vi "CompressAndUpdate(NumericArray).vi"(7 "force CVT update (false)":bool, 8 "error in":errorcluster, 9 "precision (6)":i16=6, 10 "Numeric Array":dbl[](array[numeric]), 11 "command or variable name":string) -> (0 "error out":errorcluster)   [LabVIEW 2011]
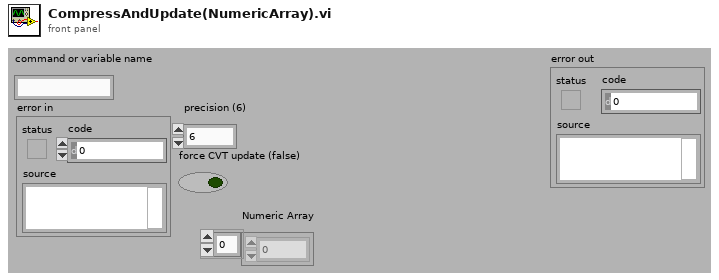
[diagram p1: front panel]
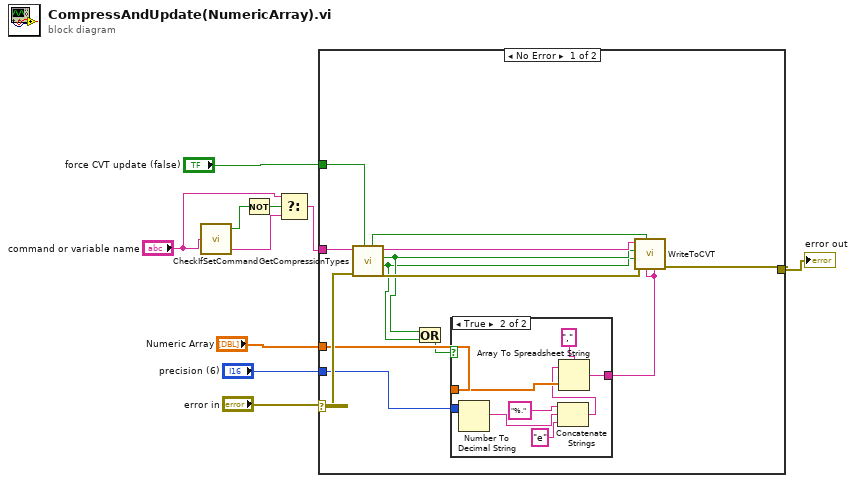
[diagram p0: block diagram]
diagram:
  n1 = call "CheckIfSetCommand.vi"("Command"="command or variable name") -> ("setCommand?"=w5:bool, "variable"=w3:string)  [unwired: 1 out]
  n2 = Not(x=w5) -> (.not. x?=w6:bool)
  n3 = Select(t="command or variable name", s=w6, f=w3) -> (s? t:f=w2:string)
  n4 = case shown="No Error" "error in" {
    selector: "error in" -> [w23 w32]
    tunnel: [w17 w32] -> w10
    tunnel: w2 -> [w18 _]
    tunnel: "Numeric Array" -> [w22 _]
    tunnel: "precision (6)" -> [w21 _]
    tunnel: "force CVT update (false)" -> [w15 _]
    frame No Error {
      n5 = call "GetCompressionTypes.vi"("force CVT update"=w15, "error in"=w23, "variable"=w18) -> ("error out"=w19:errorcluster, "non compressed"=w11:bool, "compressed"=w12:bool, "variable out"=w13:string, "force CVT update out"=w14:bool)  [unwired: 4 in]
      n6 = Or(x=w12, y=w11) -> (x .or. y?=w20:bool)
      n7 = case shown="True" w20 {
        tunnel: w22 -> [_ w30]
        tunnel: w21 -> [_ w29]
        tunnel: [_ w24] -> w16
        frame False {
        }
        frame True {
          n8 = Number To Decimal String(number=w29) -> (decimal integer string=w27:string)  [unwired: 1 in]
          n9 = Concatenate Strings("%." ("format string"), w27, "e" ("string")) -> (w25:string)
          n10 = Array To Spreadsheet String(delimiter (Tab)=",", array=w30, 3:w25) -> (spreadsheet string=w24:string)
        }
      }
      n11 = call "WriteToCVT.vi"("non compressed string"=w16, "compressed string"=w16, "force CVT update"=w14, "error in"=w19, "non compressed"=w11, "compressed"=w12, "variable"=w13) -> ("error out"=w17:errorcluster)  [unwired: 4 in]
    }
    frame Error {
    }
  }
  "error out" <- w10
